vi "MakeMap.vi"() -> (0 "error out":errorcluster, 3 "Operational Map":picture)   [LabVIEW 2014]
panel:
  out "Image Type":T1 items=["Grayscale (U8)", "Grayscale (I16)", "Grayscale (SGL)", "Complex (CSG)", "RGB (U32)", "HSL (U32)", "RGB (U64)", "Grayscale (U16)"]
  out "Map Image":T2(plugin-control)
  out "X Resolution":i32
  out "Y Resolution":i32
  out "AddressMissionMap":path
  in  "Select a Mission Map":string
  # "Can use to map pixels to feet and to pull color off map"
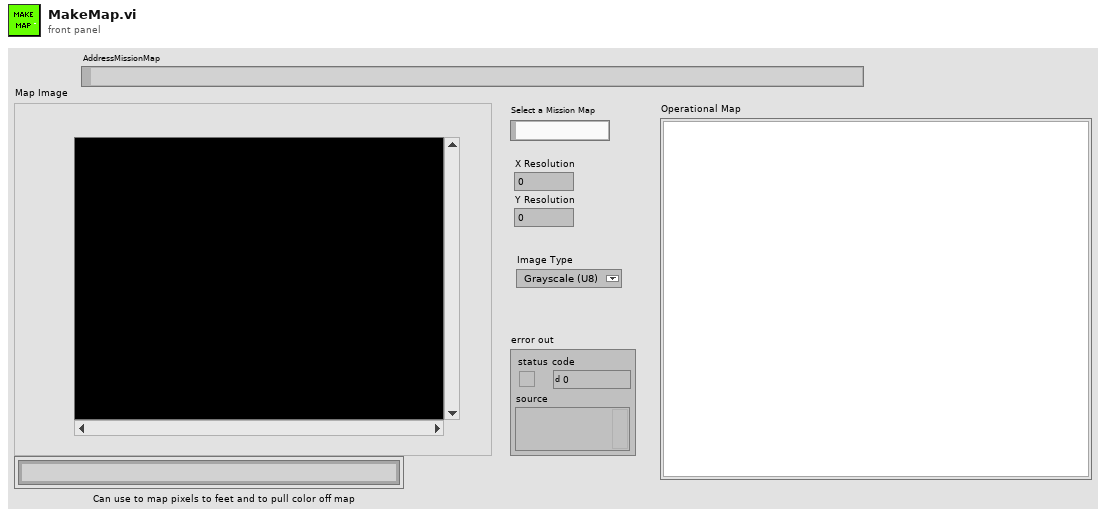
[diagram p1: front panel]
types:
  T1 = typedef "Image Type" = u32
  T2 = typedef "IMAQ Image.ctl" = refnum<image>
  T3 = typedef "imagedata.ctl" = cluster{"image type":i32, "image depth":i32, "image":u8[], "mask":u8[], "colors":u32[], "Rectangle":cluster{"left":i16, "top":i16, "right":i16, "bottom":i16}}
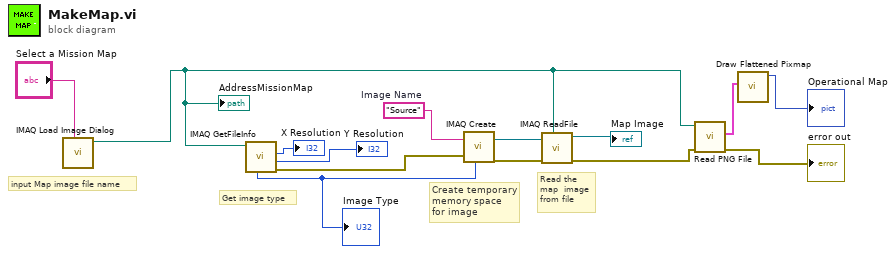
[diagram p0: block diagram]
diagram:
  w10 = "Source"  # Image Name
  # "input Map image file name"
  # "Get image type"
  # "Read the\nmap  image\nfrom file"
  # "Create temporary\nmemory space \nfor image"
  n1 = call "IMAQ Load Image Dialog"("Prompt"="Select a Mission Map") -> ("Path"=w5:path)  [unwired: 6 in, 4 out]
  "AddressMissionMap" <- w5
  n2 = call "IMAQ GetFileInfo"("File Path"=w5) -> ("error out"=w9:errorcluster, "Y Resolution"=→"Y Resolution":i32, "X Resolution"=→"X Resolution":i32, "Image Type"=w3:T1)  [unwired: 1 in, 6 out]
  "Image Type" <- w3
  n3 = call "IMAQ Create"("Image Name"=w10, "Image Type"=w3, "error in (no error)"=w9) -> ("New Image"=w8:T2, "error out"=w7:errorcluster)  [unwired: 1 in, 1 out]
  n4 = call "IMAQ ReadFile"("File Path"=w5, "error in (no error)"=w7, "Image"=w8) -> ("error out"=w2:errorcluster, "Image Out"=→"Map Image":T2)  [unwired: 2 in, 5 out]
  n5 = call <vilib>:"Read PNG File.vi"("error in (no error)"=w2, "path to PNG file"=w5) -> ("error out"=→"error out":errorcluster, "image data"=w6:T3)  [unwired: 7 in, 1 out]
  n6 = call <vilib>:"Draw Flattened Pixmap.vi"("image data"=w6) -> ("new picture"=→"Operational Map":picture)  [unwired: 8 in]
